vi "ParameterChange.vi"(2 "System":u16(ring)=1 items=["Cusp", "Positron", "Musashi"], 3 "Slow AO Qname":T1, 4 "Handler Qname":T1) -> ()   [LabVIEW 2018]
uses:
  <vilib>/NI/AMC/Message Queue.ctl
  <vilib>/NI/AMC/Message.ctl
  <vilib>/NI/Tools/Keyed Array/KeyedArray.ctl
  <vilib>/Utility/error.llb/DialogType.ctl
  ParameterSubCluster.ctl
  <vilib>/DAQmx/write.llb/DAQmx Write (Analog 1D DBL NChan 1Samp).vi
  <vilib>/NI/AMC/Read Termination Message.vi
  <vilib>/NI/AMC/Create Single Message.vi
  <vilib>/NI/AMC/Update Message Routing Info.vi
  <vilib>/DAQmx/create/channels.llb/DAQmx Create Channel (AO-Voltage-Basic).vi
  <vilib>/NI/AMC/Globals.vi
  <vilib>/DAQmx/miscellaneous.llb/DAQmx Fill In Error Info.vi
  <vilib>/NI/AMC/Send Message.vi
  <vilib>/NI/AMC/AMC.lvlib
  <vilib>/NI/Tools/Keyed Array/Tools_KeyedArray.lvlib
panel:
  in  "Array":dbl[](array[numeric])
  in  "Voltage limit for 6723":dbl=10.0 format="%#_13g"
  out "Array out":dbl[][](array[numeric])
  in  "Max sample rate (10k)":dbl=10000.0 format="%#_13g"
  in  "Ramp samples (100)":i32=100
  out "error out":errorcluster
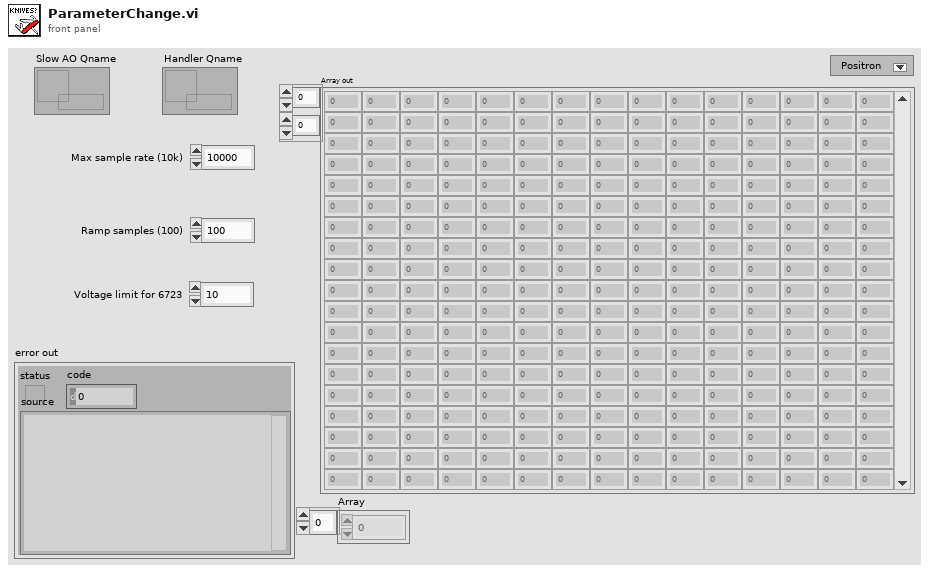
[diagram p1: front panel]
types:
  T1 = typedef "AMC.lvlib/Message Queue.ctl" = refnum<queue>
  T2 = typedef "DialogType.ctl" = u16
  T3 = typedef "ParameterSubCluster.ctl" = cluster{"ao line":string, "Duration, Gain, NewVal":dbl[]}[]
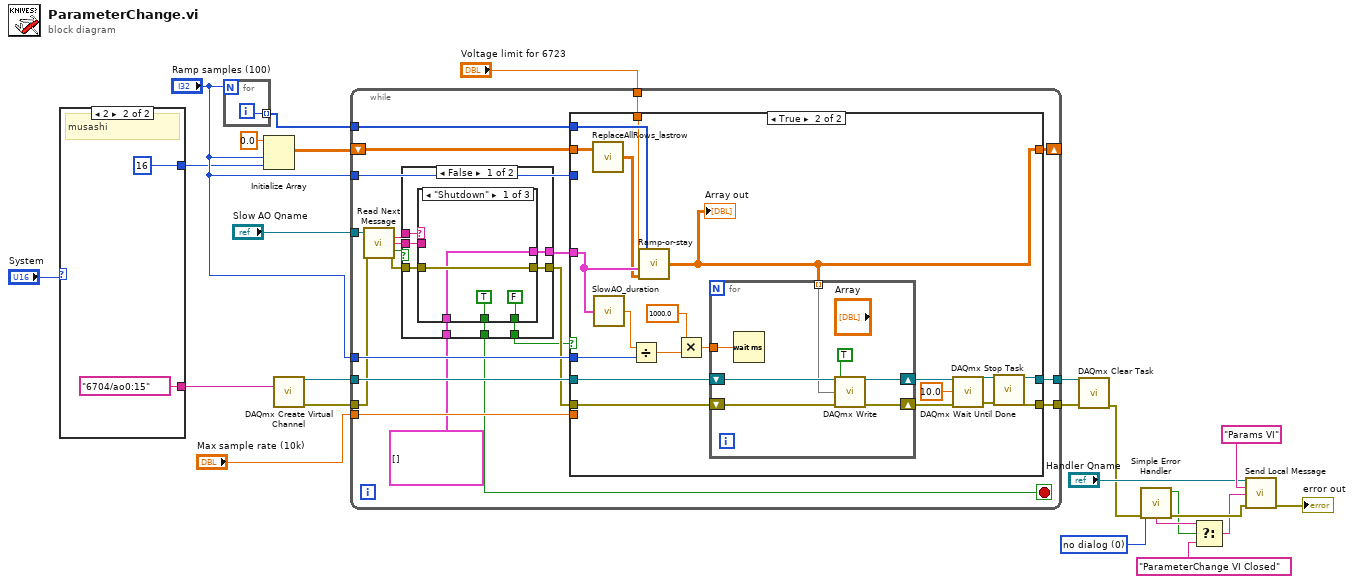
[diagram p0: block diagram]
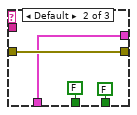
[diagram p3: hidden frame]
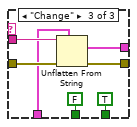
[diagram p4: hidden frame]
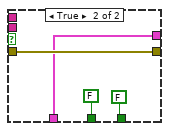
[diagram p5: hidden frame]
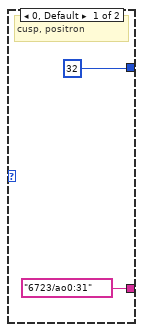
[diagram p6: hidden frame]
diagram:
  w14 = T2 0 items=["no dialog", "OK message", "continue or stop message", "OK message + warnings", "continue/stop + warnings"] ("type of dialog (OK msg:1)")
  n1 = case shown="2" "System" {
    tunnel: [tag "6723/ao0:31" ("physical channels") tag "6704/ao0:15" ("physical channels")] -> w18
    tunnel: [32 ("ao lines (32)") 16 ("ao lines (32)")] -> w9
    frame 0, Default {
      # "cusp, positron"
    }
    frame 2 {
      # "musashi"
    }
  }
  n2 = for {
    N: "Ramp samples (100)" -> [_]
    tunnel: [w29] -> w15 mode=indexing
    i -> [w29]
  }
  n3 = Initialize Array(0.0 ("element"), "Ramp samples (100)", w9) -> (w16:dbl[][])
  n4 = call-poly <vilib>:"DAQmx Create Virtual Channel.vi"("physical channels"=w18) -> ("task out"=w22:refnum<k21>, "error out"=w21:errorcluster)  [unwired: 13 in]
  n5 = while {
    shift-right: [w38] -> _
    shift-left: w16 -> [w41]
    tunnel: "Slow AO Qname" -> [w47]
    tunnel: w22 -> [w46]
    tunnel: w21 -> [w36]
    tunnel: [w45] -> w20
    tunnel: [w44] -> w19
    tunnel: "Ramp samples (100)" -> [w43]
    tunnel: "Max sample rate (10k)" -> [w42]
    tunnel: "Ramp samples (100)" -> [w40]
    tunnel: w15 -> [w39]
    tunnel: "Voltage limit for 6723" -> [w30]
    stop <- w33 stop-if-true
    n6 = call <vilib>:"Read Next Message.vi"("message queue in"=w47, "error in"=w36) -> ("message name"=w37:string, "message value"=w48:string, "timed out?"=w49:bool, "error out"=w35:errorcluster)  [unwired: 6 in, 4 out]
    n7 = case shown="False" w49 {
      tunnel: w48 -> [w88 _]
      tunnel: [w87 w105] -> w50
      tunnel: w37 -> [w86 _]
      tunnel: [w85 FALSE] -> w33
      tunnel: w35 -> [w84 w106]
      tunnel: [w83 w106] -> w34
      tunnel: T3 [] ("Slow AO Array") -> [w82 w105]
      tunnel: [w81 FALSE] -> w31
      frame False {
        n8 = case shown="\"Shutdown\"" w86 {
          tunnel: w88 -> [_ _ w103]
          tunnel: [w90 w94 w102] -> w87
          tunnel: [TRUE FALSE FALSE] -> w85
          tunnel: w84 -> [w91 w95 w100]
          tunnel: [w91 w95 w99] -> w83
          tunnel: w82 -> [w90 w94 w98]
          tunnel: [FALSE FALSE TRUE] -> w81
          frame "Shutdown" {
          }
          frame Default {
          }
          frame "Change" {
            n9 = Unflatten From String(type=w98, binary string=w103, error in (no error)=w100) -> (value=w102:T3, error out=w99:errorcluster)  [unwired: 2 in, 1 out]
          }
        }
      }
      frame True {
      }
    }
    n10 = case shown="True" w31 {
      tunnel: w50 -> [_ w64]
      tunnel: w46 -> [w51 w70]
      tunnel: w34 -> [w52 w65]
      tunnel: [w51 w61] -> w45
      tunnel: [w52 w60] -> w44
      tunnel: w43 -> [_ w68]
      tunnel: w42 -> [_ _]
      tunnel: w41 -> [w53 w67]
      tunnel: w40 -> [_ _]
      tunnel: w39 -> [_ w66]
      tunnel: [w53 w58] -> w38
      tunnel: w30 -> [_ w57]
      frame False {
        # "timed out with no command"
      }
      frame True {
        n11 = call "ReplaceAllRows_lastrow.vi"("Array in"=w67) -> ("Array out"=w59:dbl[][])  [unwired: 1 in]
        n12 = call "SlowAO_duration.vi"("Slow AO Array"=w64) -> ("Duration (s)"=w69:dbl)
        n13 = Divide(x=w69, y=w68) -> (x/y=w56:dbl)
        n14 = call "Ramp-or-stay.vi"("Array in"=w59, "Slow AO Array"=w64, "Voltage limit for 6723"=w57, "Array 2"=w66) -> ("Array"=w58:dbl[][])
        "Array out" <- w58
        n15 = Multiply(x=1000.0, y=w56) -> (x*y=w54:dbl)
        n16 = for {
          tunnel: w58 -> [w75] mode=indexing
          shift-right: [w80] -> w73
          shift-left: w65 -> [w77]
          shift-right: [w79] -> w72
          shift-left: w70 -> [w76]
          tunnel: w54 -> [w74]
          n17 = Wait (ms)(milliseconds to wait=w74) -> ()  [unwired: 1 out]
          n18 = call-poly <vilib>:"DAQmx Write.vi"("task/channels in"=w76, "auto start"=TRUE, "data"=w75, "error in"=w77) -> ("task out"=w79:refnum<k21>, "error out"=w80:errorcluster)  [unwired: 9 in, 1 out]
        }
        n19 = call <vilib>:"DAQmx Wait Until Done.vi"("task/channels in"=w72, "timeout (sec)"=10.0, "error in"=w73) -> ("task out"=w62:refnum<k21>, "error out"=w63:errorcluster)  [unwired: 11 in]
        n20 = call <vilib>:"DAQmx Stop Task.vi"("task/channels in"=w62, "error in"=w63) -> ("task out"=w61:refnum<k21>, "error out"=w60:errorcluster)  [unwired: 12 in]
      }
    }
  }
  n21 = call <vilib>:"DAQmx Clear Task.vi"("task in"=w20, "error in"=w19) -> ("error out"=w11:errorcluster)  [unwired: 13 in]
  n22 = call <vilib>:"Simple Error Handler.vi"("type of dialog (OK msg:1)"=w14, "error in (no error)"=w11) -> ("error?"=w5:bool, "error out"=w8:errorcluster, "message"=w6:string)  [unwired: 3 in, 2 out]
  n23 = Select(t=w6, s=w5, f="ParameterChange VI Closed") -> (s? t:f=w4:string)
  n24 = call <vilib>:"Send Local Message.vi"("message queue in"="Handler Qname", "message name"="Params VI", "message value"=w4, "error in"=w8) -> ("error out"=→"error out":errorcluster)  [unwired: 9 in, 2 out]
